vi "Edit DPID.vi"(8 "error in (no error)":errorcluster, 11 "Node Ptr":u64 format="%.0x") -> (0 "error out":errorcluster)   [LabVIEW 2019, in "Diagnostics Addon System Explorer.lvlib"]
uses:
  Diagnostics Addon System Explorer.lvlib
  Types/FG.Action.ctl
  SubVIs/ID.FG.vi
  SubVIs/Signals.Get.vi
  SubVIs/Type.FG.vi
  SubVIs/Frame.Convert.Name.vi
  SubVIs/Signal.FG.vi
  SubVIs/Frame.GetSignalRefs.vi
  Addon Shared/SubVIs/Constants.vi
  <vilib>/NI/NI VeriStand Advanced SysDef API/SysDef API/SysDef.Property.Set.vi
  <vilib>/NI/NI VeriStand Advanced SysDef API/_SubVIs/SysDef.Property.Set.U32.vi
  <vilib>/NI VeriStand/Custom Device API/NI VeriStand - Get Item Property.vi
  <vilib>/NI VeriStand/Custom Device API/Get Item Property (U32).vi
  <vilib>/NI/NI VeriStand Advanced SysDef API/_SubVIs/SysDef.Property.Set.U32.Array.vi
  <vilib>/NI VeriStand/Custom Device API/Get Item Property (U32 Array).vi
  <vilib>/NI VeriStand/Custom Device Tools/Custom Device Utility Library/NI VeriStand - Search for All Items by GUID.vi
  <vilib>/NI VeriStand/Custom Device Tools/Custom Device Utility Library/NI VeriStand - Search for Item by GUID.vi
  <vilib>/NI VeriStand/Custom Device API/NI VeriStand - Get Item Data.vi
  <vilib>/NI/NI VeriStand Advanced SysDef API/_SubVIs/SysDef.Property.Set.DBL.vi
  <vilib>/NI/NI VeriStand Advanced SysDef API/_SubVIs/SysDef.Property.Set.String.vi
  <vilib>/NI VeriStand/Custom Device API/Get Item Property (Double).vi
  <vilib>/NI VeriStand/Custom Device API/Get Item Property (String).vi
  <vilib>/NI VeriStand/Custom Device API/NI VeriStand - Get Custom Device Channel Data.vi
  <vilib>/NI VeriStand/Custom Device Tools/Custom Device Utility Library/Custom Device Utility Library.lvlib
  Addon Shared/Diagnostics Addon Shared.lvlib
  <vilib>/NI VeriStand/Custom Device API/Custom Device API.lvlib
panel:
  in  "Tag":string
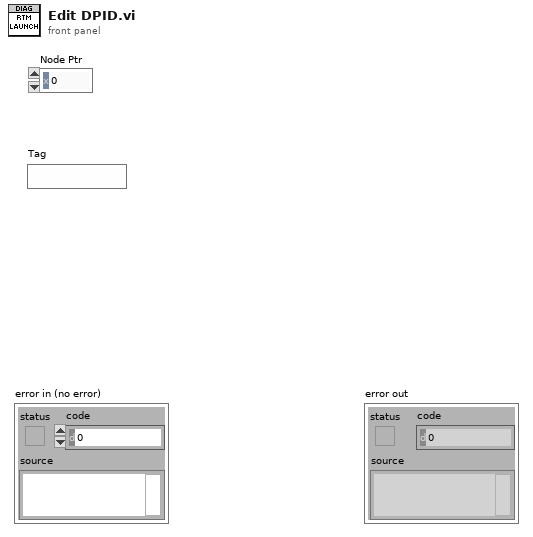
[diagram p1: front panel]
types:
  T1 = typedef "Diagnostics Addon System Explorer.lvlib/FG.Action.ctl" = enum16{"Get", "Set"}
  T2 = typedef "Diagnostics Addon Shared.lvlib/DPID.ctl" = cluster{"DPID ID":u8, "Speed":T3, "PIDs":u16[]}
  T3 = typedef "Diagnostics Addon Shared.lvlib/DPID.Rate.ctl" = enum16{"Slow", "Medium", "Fast"}
  T4 = typedef "Custom Device API.lvlib/Custom Device Item Ref.ctl" = u64
  T5 = typedef "Diagnostics Addon System Explorer.lvlib/Frame.Export.ctl" = cluster{"Name":string, "ID":u32, "Signals":T6[]}
  T6 = typedef "Diagnostics Addon Shared.lvlib/Signal.ctl" = cluster{"Start Bit":u32, "Length":u32, "Scaling Factor":dbl, "Scaling Offset":dbl, "Minimum":dbl, "Maximum":dbl, "Data Type":u32, "Byte Order":u32, "Default Value":dbl, "Name":string, "Units":string}
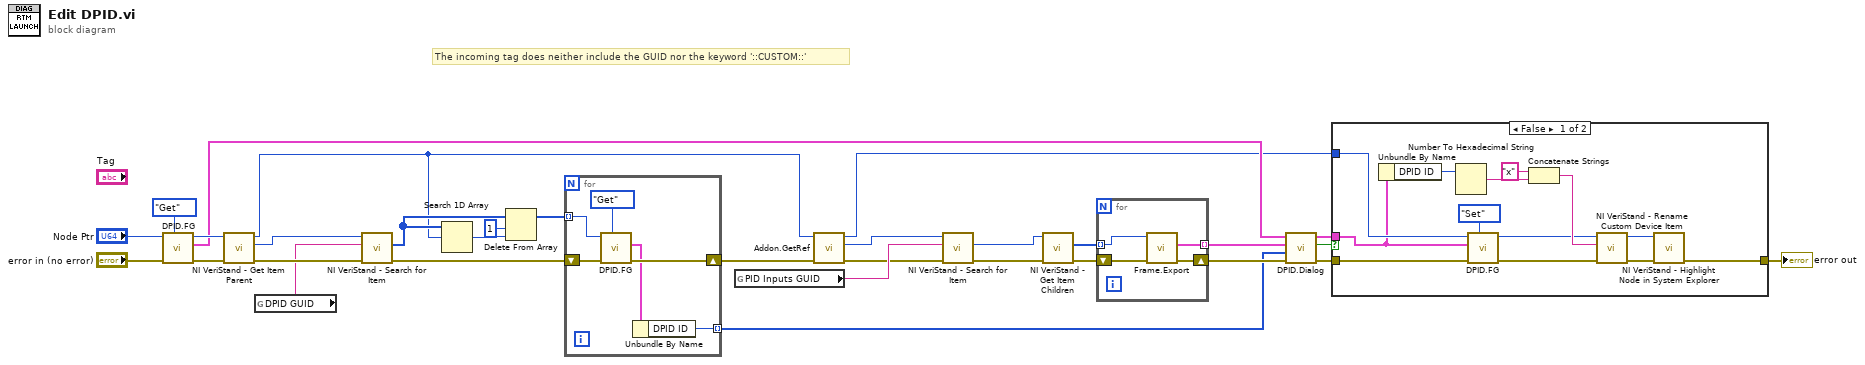
[diagram p0: block diagram]
diagram:
  # "The incoming tag does neither include the GUID nor the keyword '::CUSTOM::'"
  n1 = call "DPID.FG.vi"("Action"=FG.Action."Get", "error in (no error)"="error in (no error)", "Device Item Ref in"="Node Ptr") -> ("error out"=w15:errorcluster, "DPID"=w7:T2, "Device Item Ref out"=w18:T4)  [unwired: 6 in]
  n2 = call <vilib>:"NI VeriStand - Get Item Parent.vi"("error in (no error)"=w15, "Item Ref in"=w18) -> ("error out"=w14:errorcluster, "Parent Ref"=w16:T4, "Item Ref out"=w6:T4)  [unwired: 6 in, 1 out]
  n3 = global read "Constants.vi" "DPID GUID"() -> (w1:string)
  n4 = call-poly <vilib>:"NI VeriStand - Search for Item.vi"("error in"=w14, "Item GUID"=w1, "Section Ref in"=w16) -> ("error out"=w28:errorcluster, "Item Refs"=w11:T4[])  [unwired: 5 in, 2 out]
  n5 = Search 1D Array(1D array=w11, element=w6) -> (index of element=w12:i32)  [unwired: 1 in]
  n6 = Delete From Array(array=w11, length=1, index=w12) -> (array with subset deleted=w10:T4[])  [unwired: 1 out]
  n7 = for {
    tunnel: w10 -> [w37] mode=indexing
    shift-right: [w35] -> w2
    shift-left: w28 -> [w36]
    tunnel: [w33] -> w24 mode=indexing
    n8 = call "DPID.FG.vi"("Action"=FG.Action."Get", "error in (no error)"=w36, "Device Item Ref in"=w37) -> ("error out"=w35:errorcluster, "DPID"=w34:T2)  [unwired: 6 in, 1 out]
    n9 = Unbundle By Name(w34) -> ("DPID ID"=w33:u8)
  }
  n10 = global read "Constants.vi" "PID Inputs GUID"() -> (w31:string)
  n11 = call "Addon.GetRef.vi"("error in (no error)"=w2, "Node Ptr"=w6) -> ("error out"=w3:errorcluster, "Addon Ref"=w5:T4, "Node Ptr"=w4:T4)  [unwired: 7 in]
  n12 = call-poly <vilib>:"NI VeriStand - Search for Item.vi"("error in"=w3, "Item GUID"=w31, "Section Ref in"=w5) -> ("error out"=w30:errorcluster, "Item Ref"=w29:T4)  [unwired: 5 in, 2 out]
  n13 = call <vilib>:"NI VeriStand - Get Item Children.vi"("error in (no error)"=w30, "Item Ref in"=w29) -> ("error out"=w27:errorcluster, "Child Refs"=w26:T4[])  [unwired: 6 in, 2 out]
  n14 = for {
    tunnel: w26 -> [w41] mode=indexing
    tunnel: [w38] -> w8 mode=indexing
    shift-right: [w39] -> w25
    shift-left: w27 -> [w40]
    n15 = call "Frame.Export.vi"("error in (no error)"=w40, "Item Ref in"=w41) -> ("error out"=w39:errorcluster, "Frame"=w38:T5)  [unwired: 7 in, 1 out]
  }
  n16 = call "DPID.Dialog.vi"("error in (no error)"=w25, "Existing DPIDs"=w24, "Existing PIDs"=w8, "DPID"=w7) -> ("error out"=w21:errorcluster, "Cancel PID?"=w23:bool, "DPID"=w22:T2)  [unwired: 5 in]
  n17 = case shown="False" w23 {
    tunnel: w22 -> [w42 _]
    tunnel: w21 -> [w53 w55]
    tunnel: [w44 w55] -> w20
    tunnel: w4 -> [w54 _]
    frame False {
      n18 = Unbundle By Name(w42) -> ("DPID ID"=w47:u8)
      n19 = Number To Hexadecimal String(2:w47) -> (0:w50:string)  [unwired: 1 in]
      n20 = call "DPID.FG.vi"("Action"=FG.Action."Set", "error in (no error)"=w53, "DPID"=w42, "Device Item Ref in"=w54) -> ("error out"=w49:errorcluster, "Device Item Ref out"=w48:T4)  [unwired: 5 in, 1 out]
      n21 = Concatenate Strings("x" ("element"), w50) -> (w52:string)
      n22 = call <vilib>:"NI VeriStand - Rename Custom Device Item.vi"("error in (no error)"=w49, "New Name"=w52, "Item Ref in"=w48) -> ("error out"=w45:errorcluster, "Item Ref out"=w46:T4)  [unwired: 1 in, 6 out]
      n23 = call <vilib>:"NI VeriStand - Highlight Node in System Explorer.vi"("error in (no error)"=w45, "Item Ref in"=w46) -> ("error out"=w44:errorcluster)  [unwired: 8 in, 1 out]
    }
    frame True {
    }
  }
  "error out" <- w20
